vi "StructuredDataToVariant.vi"(7 "Data Type":variant, 8 "error in (no error)":errorcluster, 10 "StructuredData":variant, 11 "BlueTOMLSerializer in":refnum<class "BlueTOMLSerializer.lvclass">) -> (0 "error out":errorcluster, 2 "Variant":variant, 3 "BlueTOMLSerializer out":refnum<class "BlueTOMLSerializer.lvclass">)   [LabVIEW 2019, in "BlueTOMLSerializer.lvlib" / "BlueTOMLSerializer.lvclass"]
uses:
  BlueTOMLSerializer.lvclass
  C:/Program Files (x86)/National Instruments/LabVIEW 2019/user.lib/Blue Origin/BlueSerialization/BlueSerializer/BlueSerializer.lvclass
  StructuredData.ctl
  Support/TOML Value.ctl
  BlueTOMLSerializer.lvlib
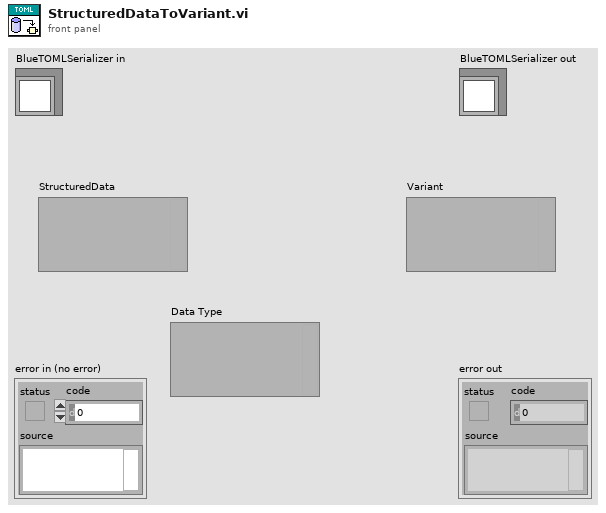
[diagram p1: front panel]
types:
  T1 = typedef "BlueTOMLSerializer.lvlib/BlueTOMLSerializer.lvclass/StructuredData.ctl" = cluster{"TOML Value":T2}
  T2 = typedef "BlueTOMLSerializer.lvlib/TOML Value.ctl" = cluster{"\\type":enum16{"Table", "Array", "String", "Integer", "Float", "Boolean", "Offset Date-Time", "Local Date-Time", "Local Date", "Local Time"}, "ÿýÿýÿýÿýÿýÿþÿýÿýÿý%LV-TOML.lvlib:TOML Key-Value Pair.ctlÿýÿýÿýÿýÿýÿþÿýÿýÿýLV-TOML.lvlib:TOML Value.ctl$":variant}
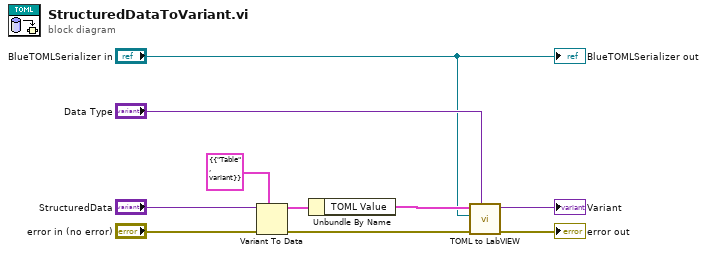
[diagram p0: block diagram]
diagram:
  n1 = Variant To Data(error in="error in (no error)", type=T1 {"TOML Value"={"\\type"=enum."Table", "ÿýÿýÿýÿýÿýÿþÿýÿýÿý%LV-TOML.lvlib:TOML Key-Value Pair.ctlÿýÿýÿýÿýÿýÿþÿýÿýÿýLV-TOML.lvlib:TOML Value.ctl$"=variant}} ("Cluster"), Variant="StructuredData") -> (data=w8:T1, error out=w3:errorcluster)
  n2 = Unbundle By Name(w8) -> ("TOML Value"=w7:T2)
  n3 = call "TOML to LabVIEW.vi"("Default Value"="Data Type", "error in (no error)"=w3, "BlueSerializer in"="BlueTOMLSerializer in", "TOML Value"=w7) -> ("error out"=→"error out":errorcluster, "LV Value"=→"Variant":variant)  [unwired: 6 in]
  "BlueTOMLSerializer out" <- "BlueTOMLSerializer in"
